vi "MicroBlaze-Tester.vi"() -> ()   [LabVIEW 2017]
doc: "Use this template to build a producer/consumer design pattern with events to produce queue items. Use this design pattern instead of the User Interface Event Handler pattern for user interfaces when you want to execute code asynchronously in response to an event without slowing the user interface responsiveness."
uses:
  MicroBlaze.States.ctl
  FpgaInterface/FpgaInterface.lvclass
panel:
  in  "AXI_STR_RXD_tkeep":fxp<+,4,4>=15.0 format="%.0b"
  out "Debug Probe 2":u64[](array[numeric]) format="%.0x"
  in  "Read Debug Probe 2":bool
  out "Debug Probe":u64[](array[numeric]) format="%.0x"
  in  "Read Debug Probe 1":bool
  out "FIFO #2 Read":u32[](array[numeric]) format="%.0x"
  in  "FIFO #2 Write":u64[](array[numeric])=[2289526357, 1144201745, 2864434397, 4009689105] format="%.0x"
  in  "Read from FIFO #2":bool
  in  "Write to FIFO #2":bool
  out "error out":errorcluster
  in  "error in (no error)":errorcluster
  in  "Write all GPIO":bool
  in  "GPIO #2":u32=4
  in  "GPIO #1":u32=3
  out "FIFO Read":u32[](array[numeric]) format="%.0x"
  out "GPIO #2":u32 format="%.0x"
  out "GPIO #1":u32 format="%.0x"
  in  "FIFO #1 Write":u32[](array[numeric])=[305419896, 2596069104, 287454020, 1432778632] format="%.0x"
  in  "Read from FIFO #1":bool
  in  "Write to FIFO #1":bool
  out "Status":string="Open FPGA Called\r\nWrite to FIFO #1\r\nRead from FIFO #3\r\nClosing FPGA\r\n"
  in  "Read all GPIO":bool
  in  "stop":bool
  # "FIFO #1 - Populate FIFO Write\nClick \"Write to FIFO #1\""
  # "FIFO #2 - Populate FIFO Write\nClick \"Write to FIFO #2"
  # "General Purose IO\nValues in Controls will be read by\nMicroBlaze and the same number\ntimes 2 will be written out to the\ncorresponding channel"
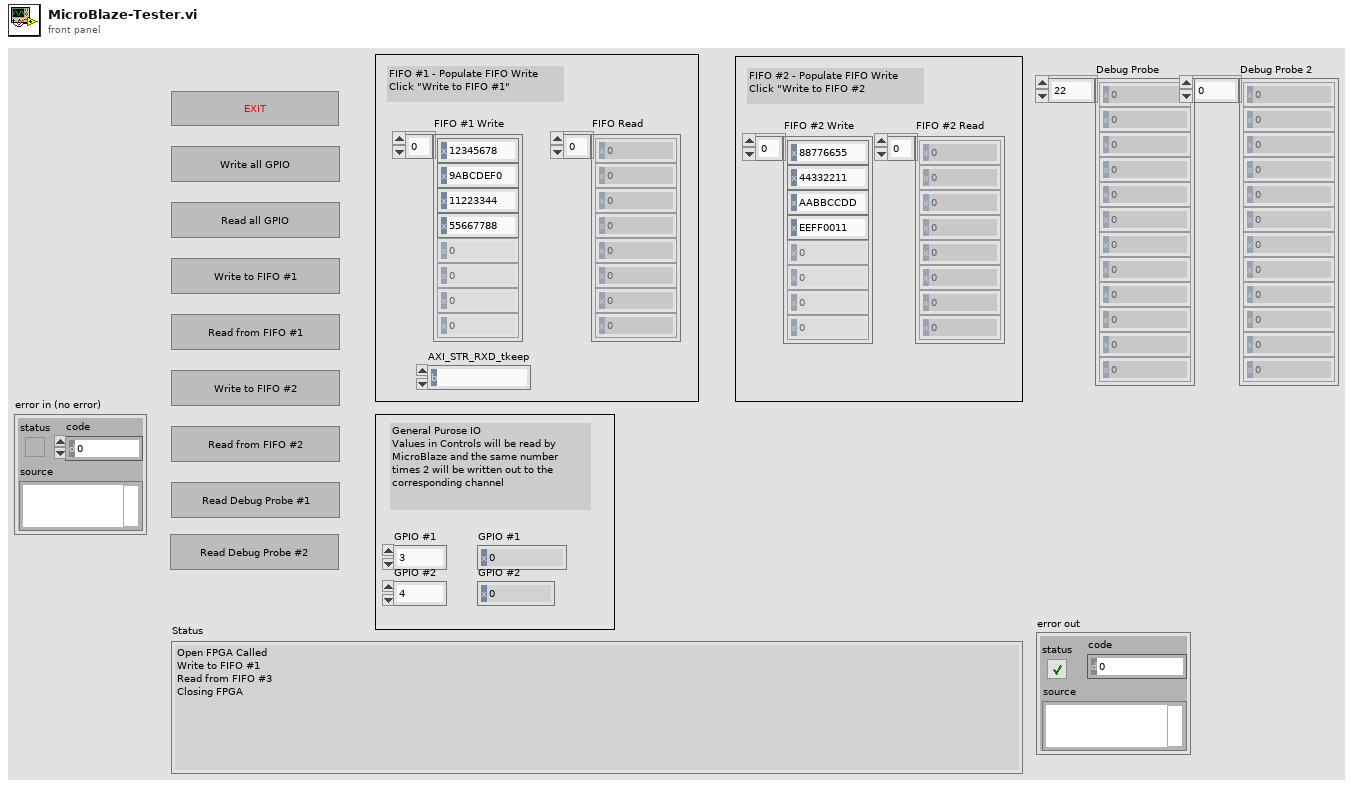
[diagram p1: front panel]
types:
  T1 = typedef "MicroBlaze.States.ctl" = enum16{"Open FPGA", "Write to GPIO", "Read all GPIO", "Write to Fifo #1", "Read from Fifo #1", "Write to Fifo #2", "Read from Fifo #2", "Read Debug Probe #1", "Read Debug Probe #2", "Close FPGA"}
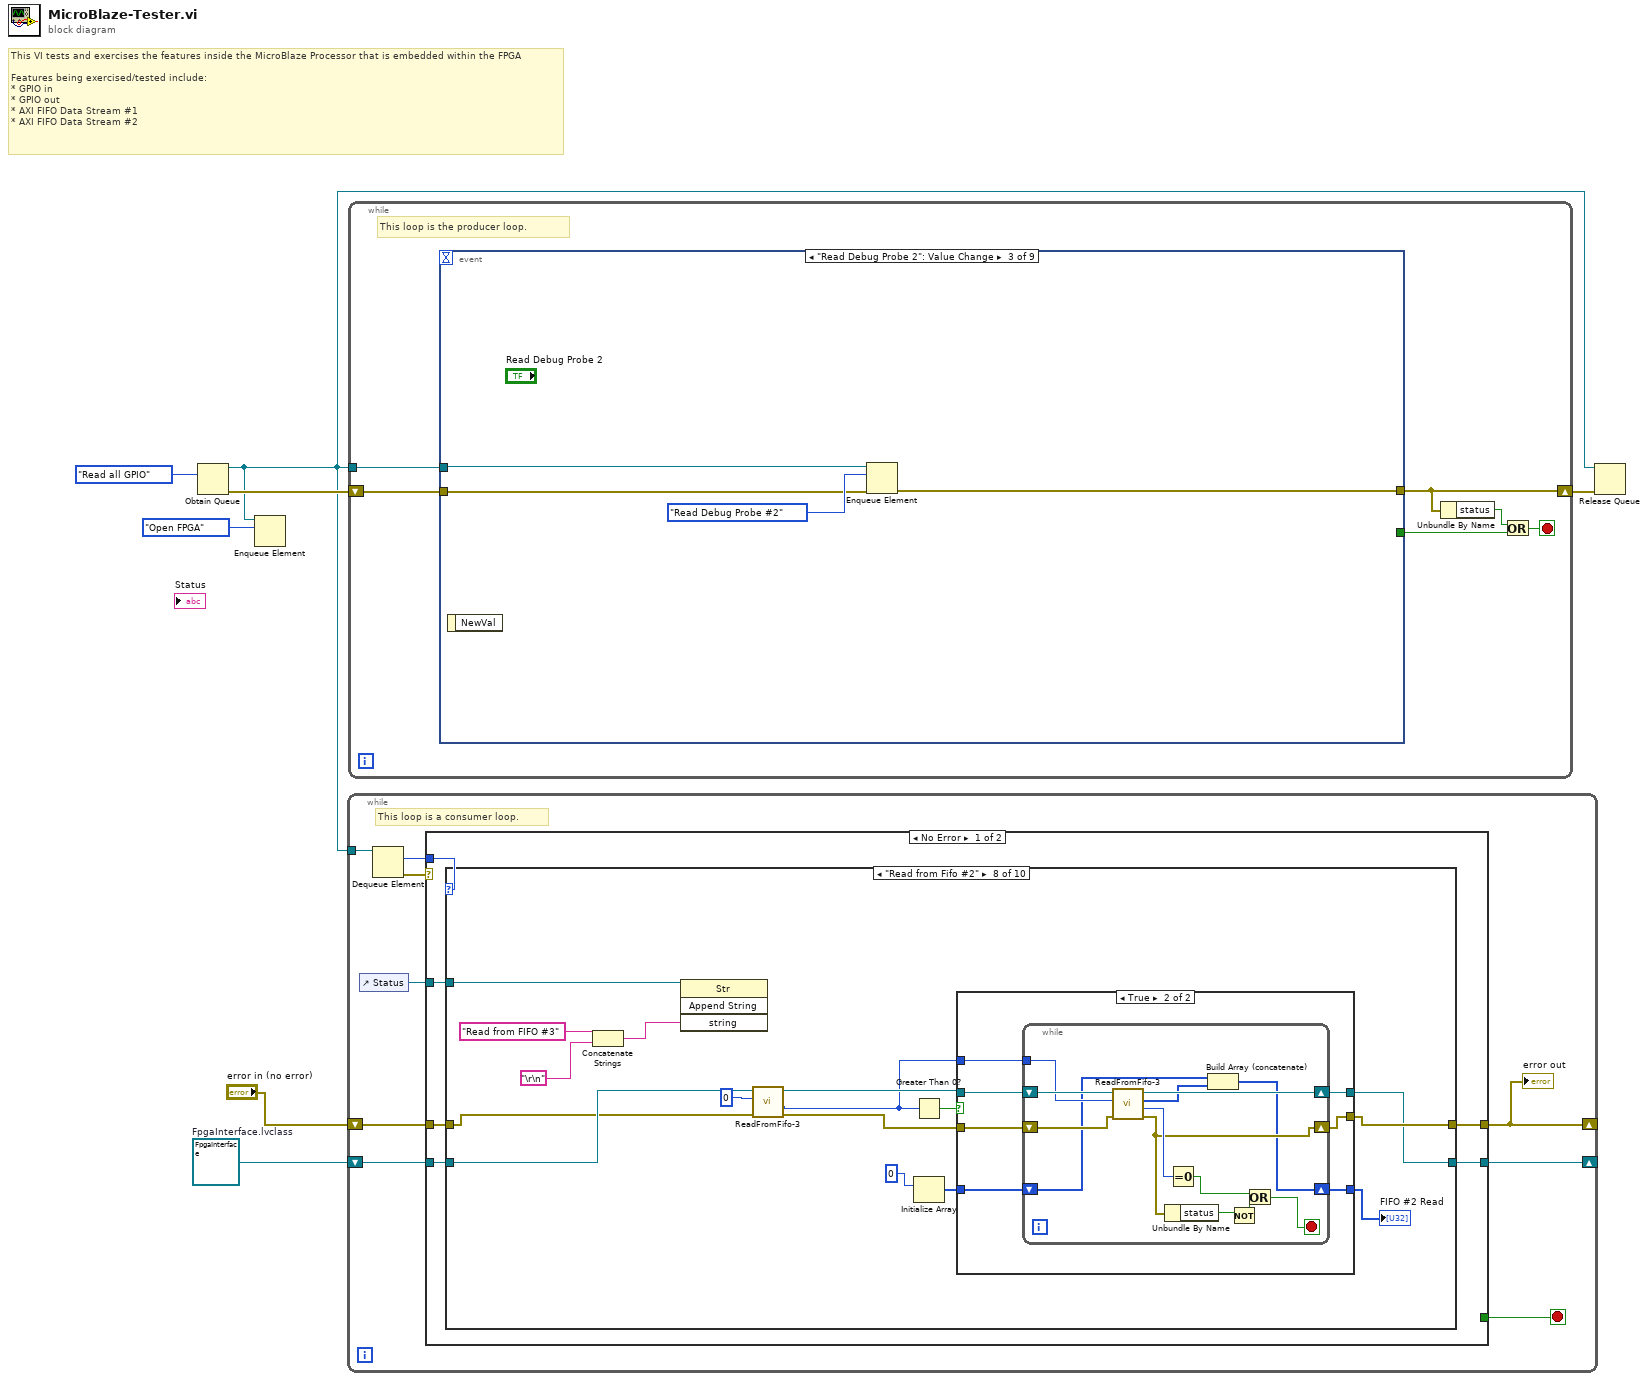
[diagram p0: block diagram]
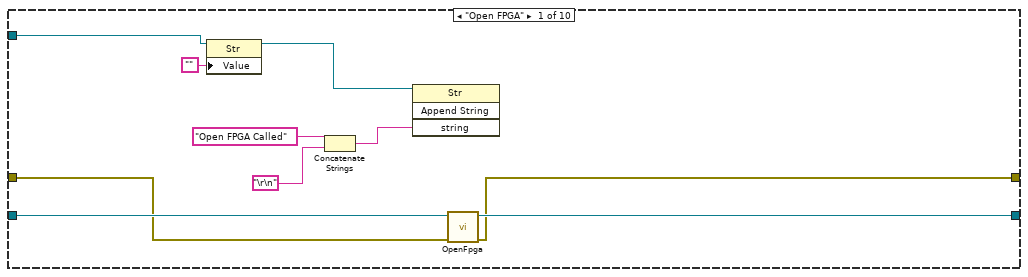
[diagram p2: hidden frame]
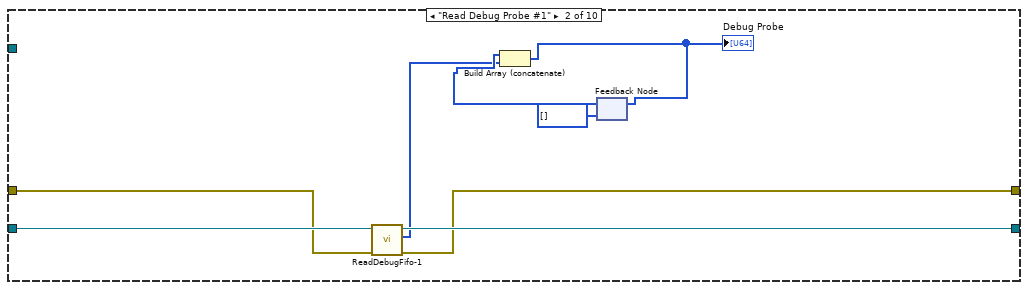
[diagram p3: hidden frame]
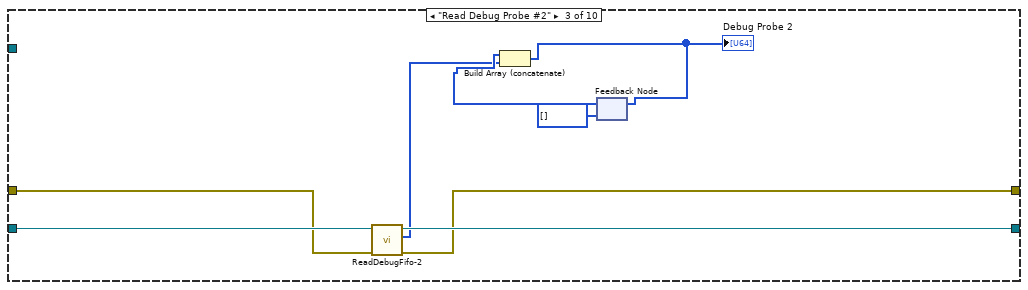
[diagram p4: hidden frame]
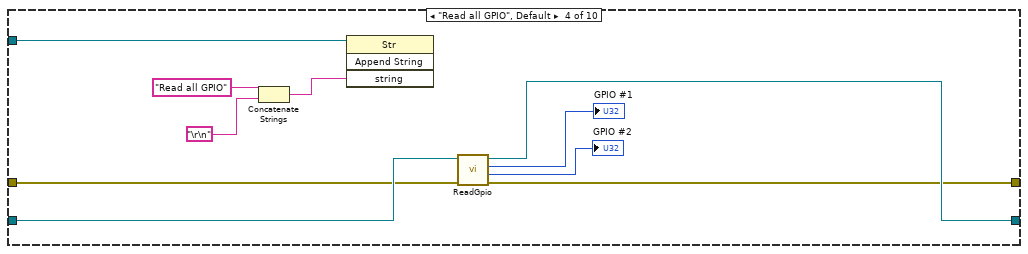
[diagram p5: hidden frame]
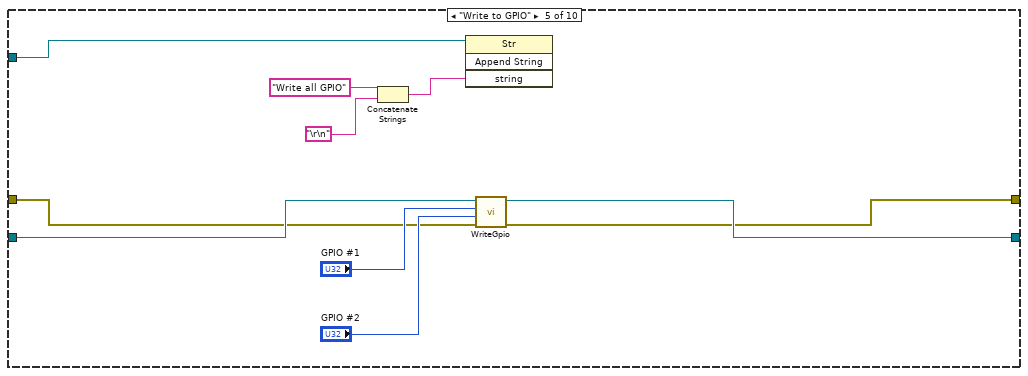
[diagram p6: hidden frame]
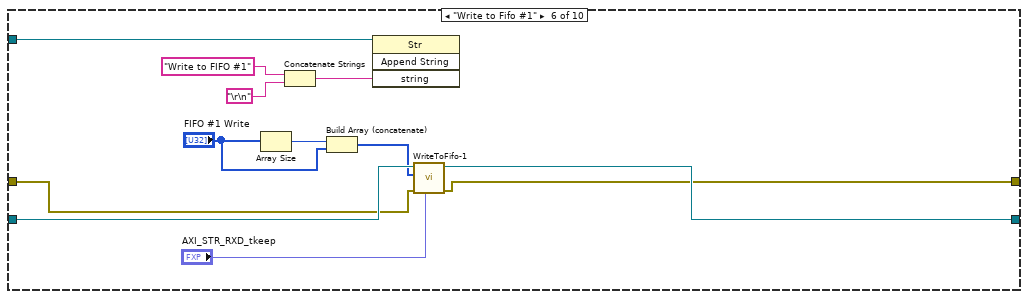
[diagram p7: hidden frame]
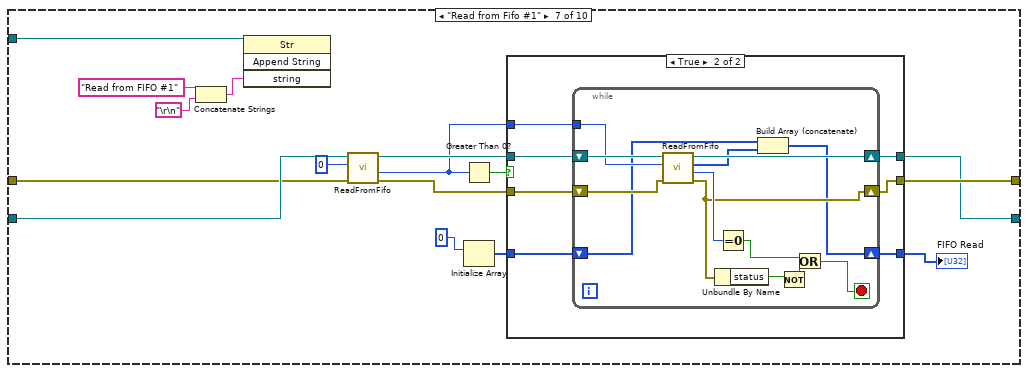
[diagram p8: hidden frame]
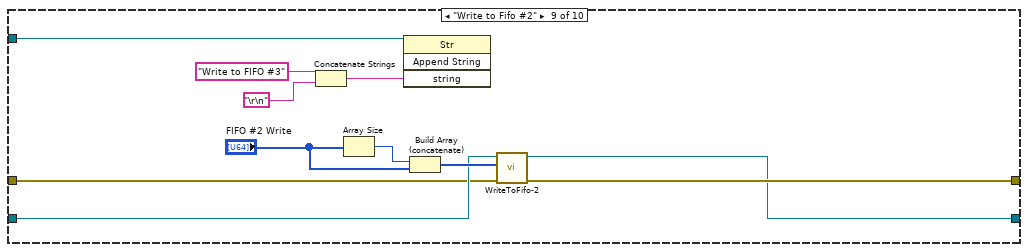
[diagram p11: hidden frame]
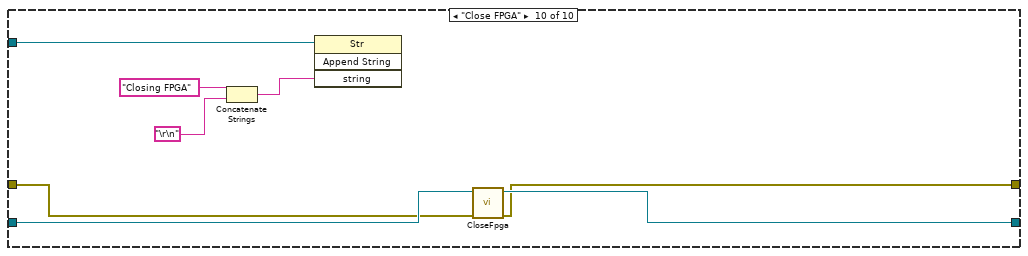
[diagram p12: hidden frame]
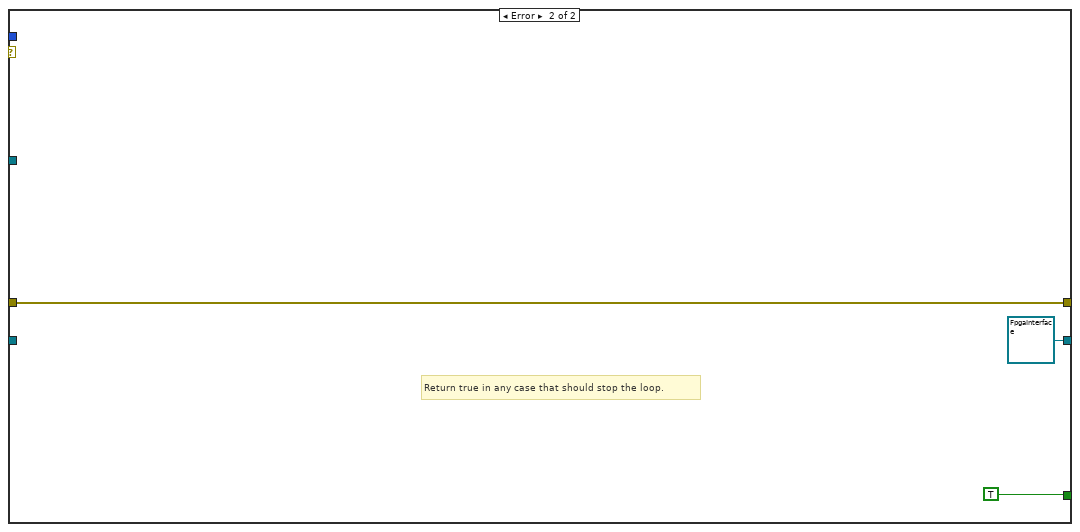
[diagram p13: hidden frame]
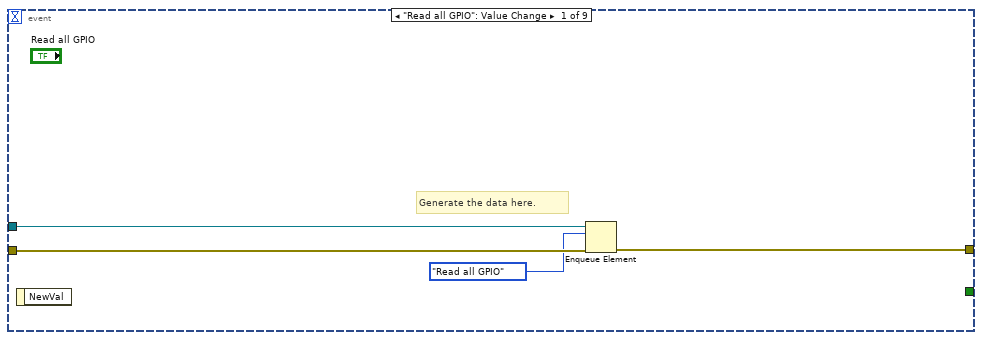
[diagram p14: hidden frame]
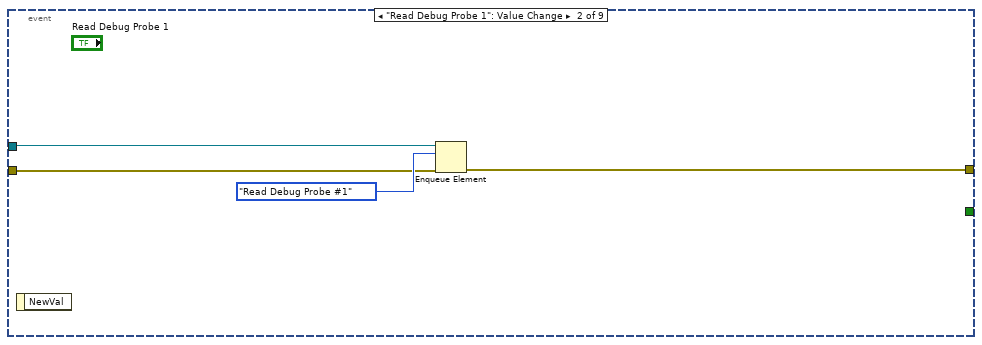
[diagram p15: hidden frame]
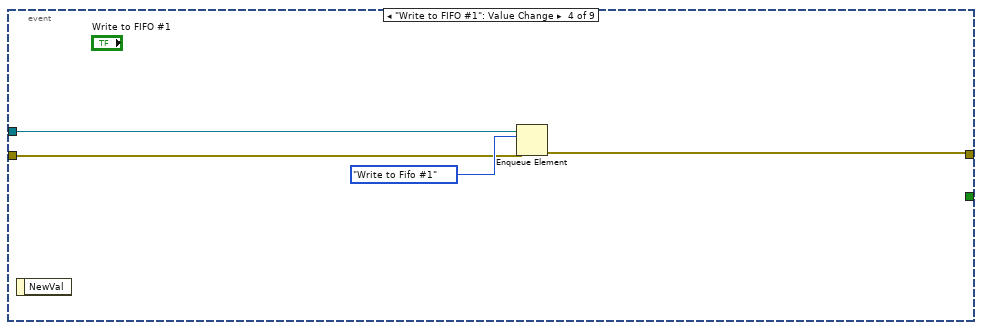
[diagram p16: hidden frame]
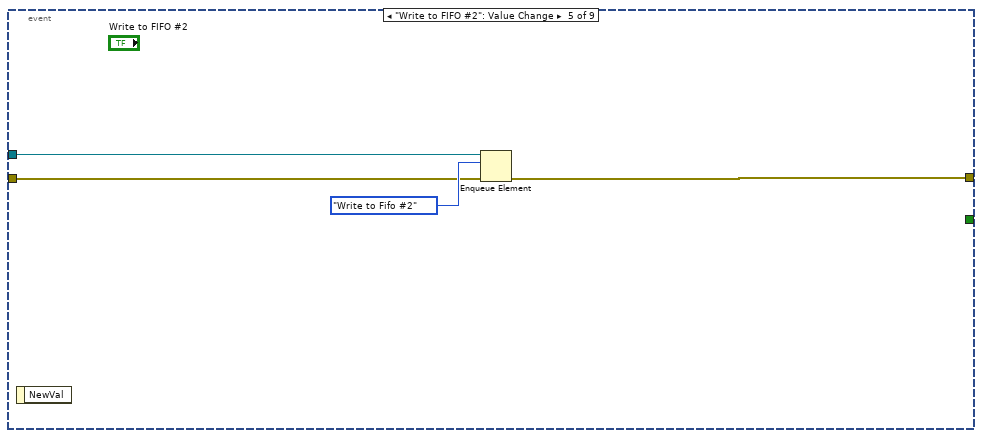
[diagram p17: hidden frame]
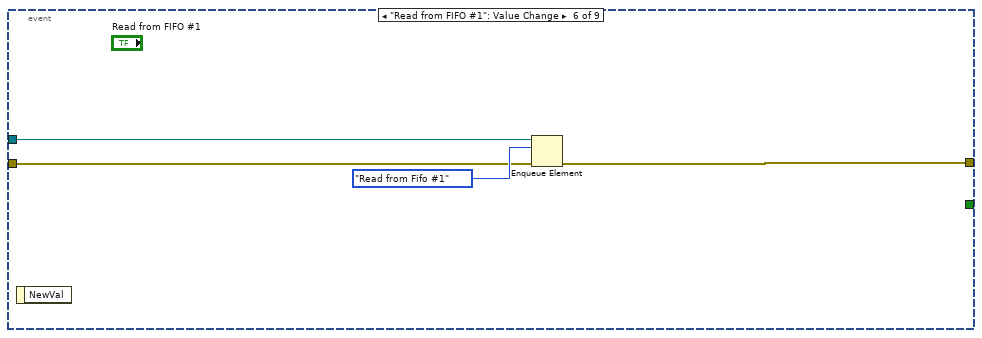
[diagram p18: hidden frame]
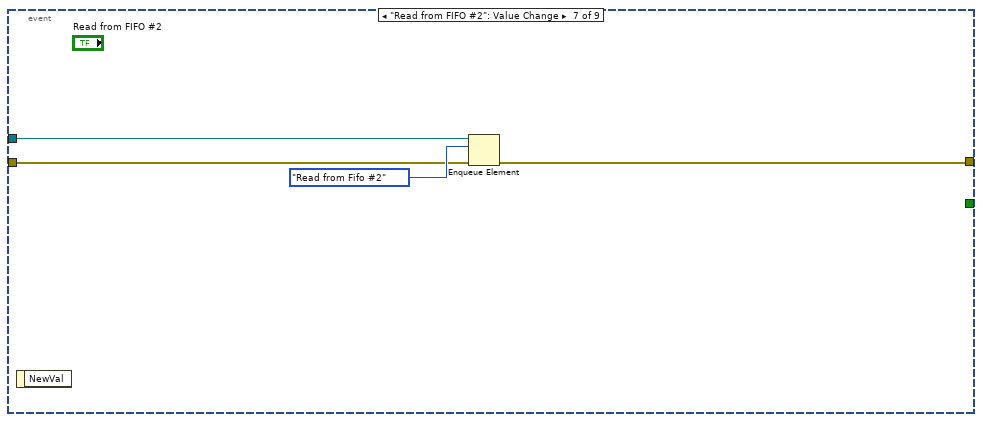
[diagram p19: hidden frame]
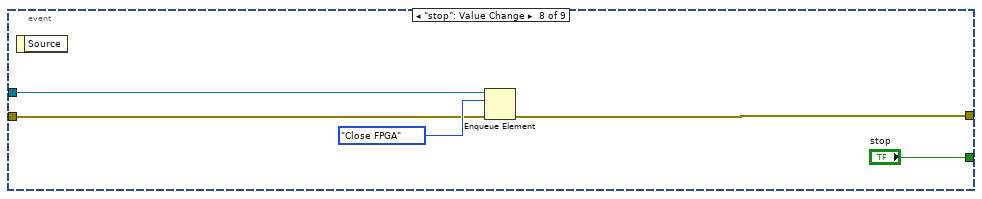
[diagram p20: hidden frame]
diagram:
  w2 = refnum<class "FpgaInterface.lvclass"> refnum  # FpgaInterface.lvclass
  # "This VI tests and exercises the features inside the MicroBlaze Processor that is embedded within the FPGA\n\nFeatures being exercised/tested include:\n* GPIO in\n* GPIO out\n* AXI FIFO Data Stream #1\n* AXI FIFO Data Stream #2"
  n1 = Obtain Queue(element data type=MicroBlaze.States."Read all GPIO" ("Events 2")) -> (queue out=w4:refnum<queue>, error out=w7:errorcluster)  [unwired: 4 in, 1 out]
  n2 = Enqueue Element(queue=w4, element=MicroBlaze.States."Open FPGA" ("Events 2")) -> ()  [unwired: 2 in, 3 out]
  n3 = while {
    tunnel: w4 -> [w16]
    shift-right: [w9] -> _
    shift-left: "error in (no error)" -> [w10]
    shift-right: [w8] -> _
    shift-left: w2 -> [w11]
    stop <- w13 stop-if-true
    # "This loop is a consumer loop."
    n4 = control-ref of="Status"() -> (w12:refnum<vi>)
    n5 = Dequeue Element(queue=w16) -> (element=w14:T1, error out=w15:errorcluster)  [unwired: 2 in, 2 out]
    n6 = case shown="No Error" w15 {
      tunnel: w14 -> [w22 _]
      tunnel: [_ TRUE] -> w13
      tunnel: w12 -> [w21 _]
      tunnel: w11 -> [w20 _]
      tunnel: [w19 refnum<class "FpgaInterface.lvclass"> refnum ("FpgaInterface out")] -> w8
      tunnel: w10 -> [w18 w178]
      tunnel: [w17 w178] -> w9
      frame No Error {
        n7 = case shown="\"Read from Fifo #2\"" w22 {
          tunnel: w21 -> [w27 _ _ w55 w65 w77 w93 w132 w166 w174]
          tunnel: w20 -> [w26 w40 w48 w54 w64 w76 w92 w131 w162 w173]
          tunnel: [w25 w38 w46 w51 w61 w75 w84 w120 w159 w172] -> w19
          tunnel: w18 -> [w24 w39 w47 w50 w60 w71 w90 w129 w161 w171]
          tunnel: [w23 w37 w45 w49 w59 w70 w85 w121 w160 w170] -> w17
          frame "Open FPGA" {
            n8 = property class="Str"(reference=w27, "Value"="") -> (reference out=w31:refnum<vi>)  [unwired: 1 in, 1 out]
            n9 = Concatenate Strings("Open FPGA Called" ("string"), "\r\n") -> (w29:string)
            n10 = invoke class="Str" method="Append String"(reference=w31, "string"=w29) -> ()  [unwired: 2 in, 4 out]
            n11 = call-dynamic "OpenFpga.vi"("error in (no error)"=w24, "FpgaInterface in"=w26) -> ("error out"=w23:errorcluster, "FpgaInterface out"=w25:refnum<class "FpgaInterface.lvclass">)  [unwired: 8 in]
          }
          frame "Read Debug Probe #1" {
            n12 = call-dynamic "ReadDebugFifo-1.vi"("error in (no error)"=w39, "FpgaInterface in"=w40) -> ("error out"=w37:errorcluster, "Data"=w35:u32[], "FpgaInterface out"=w38:refnum<class "FpgaInterface.lvclass">)  [unwired: 7 in]
            n13 = feedback #1(u64[] []) -> (w36:u64[])
            n14 = Build Array (concatenate)(w36, w35) -> (w34:u64[])
            "Debug Probe" <- w34
            n15 = feedback-in #1(w34) -> ()
          }
          frame "Read Debug Probe #2" {
            n16 = call-dynamic "ReadDebugFifo-2.vi"("error in (no error)"=w47, "FpgaInterface in"=w48) -> ("error out"=w45:errorcluster, "Data"=w43:u32[], "FpgaInterface out"=w46:refnum<class "FpgaInterface.lvclass">)  [unwired: 7 in]
            n17 = feedback #2(u64[] []) -> (w44:u64[])
            n18 = Build Array (concatenate)(w44, w43) -> (w42:u64[])
            "Debug Probe 2" <- w42
            n19 = feedback-in #2(w42) -> ()
          }
          frame "Read all GPIO", Default {
            n20 = Concatenate Strings("Read all GPIO" ("string"), "\r\n") -> (w57:string)
            n21 = invoke class="Str" method="Append String"(reference=w55, "string"=w57) -> ()  [unwired: 2 in, 4 out]
            n22 = call-dynamic "ReadGpio.vi"("error in (no error)"=w50, "FpgaInterface in"=w54) -> ("error out"=w49:errorcluster, "GPIO #2 out"=→"GPIO #2":u32, "GPIO #1 out"=→"GPIO #1":u32, "FpgaInterface out"=w51:refnum<class "FpgaInterface.lvclass">)  [unwired: 6 in]
          }
          frame "Write to GPIO" {
            n23 = Concatenate Strings("Write all GPIO" ("string"), "\r\n") -> (w67:string)
            n24 = invoke class="Str" method="Append String"(reference=w65, "string"=w67) -> ()  [unwired: 2 in, 4 out]
            n25 = call-dynamic "WriteGpio.vi"("error in (no error)"=w60, "GPIO #2 in"="GPIO #2", "GPIO #1 in"="GPIO #1", "FpgaInterface in"=w64) -> ("error out"=w59:errorcluster, "FpgaInterface out"=w61:refnum<class "FpgaInterface.lvclass">)  [unwired: 6 in]
          }
          frame "Write to Fifo #1" {
            n26 = Array Size(array="FIFO #1 Write") -> (size(s)=w74:i32)
            n27 = Concatenate Strings("Write to FIFO #1" ("string"), "\r\n") -> (w79:string)
            n28 = Build Array (concatenate)(w74, "FIFO #1 Write") -> (w72:u32[])
            n29 = invoke class="Str" method="Append String"(reference=w77, "string"=w79) -> ()  [unwired: 2 in, 4 out]
            n30 = call-dynamic "WriteToFifo-1.vi"("AXI_STR_RXD_tkeep"="AXI_STR_RXD_tkeep", "error in (no error)"=w71, "Data"=w72, "FpgaInterface in"=w76) -> ("error out"=w70:errorcluster, "FpgaInterface out"=w75:refnum<class "FpgaInterface.lvclass">)  [unwired: 6 in]
          }
          frame "Read from Fifo #1" {
            n31 = Concatenate Strings("Read from FIFO #1" ("string"), "\r\n") -> (w95:string)
            n32 = invoke class="Str" method="Append String"(reference=w93, "string"=w95) -> ()  [unwired: 2 in, 4 out]
            n33 = call-dynamic "ReadFromFifo.vi"("error in (no error)"=w90, "Number of Elements"=u32 0, "FpgaInterface in"=w92) -> ("error out"=w87:errorcluster, "Elements Remaining"=w86:u32, "FpgaInterface out"=w88:refnum<class "FpgaInterface.lvclass">)  [unwired: 5 in, 1 out]
            n34 = Greater Than 0?(x=w86) -> (x > 0?=w89:bool)
            n35 = Initialize Array(u32 0) -> (w82:u32[])  [unwired: 1 in]
            n36 = case shown="True" w89 {
              tunnel: w88 -> [w97 w106]
              tunnel: w87 -> [w98 w105]
              tunnel: w86 -> [_ w104]
              tunnel: [w98 w103] -> w85
              tunnel: [w97 w102] -> w84
              tunnel: w82 -> [w99 w101]
              tunnel: [w99 w100] -> w81
              frame False {
              }
              frame True {
                n37 = while {
                  tunnel: w104 -> [w117]
                  shift-right: [w111] -> w102
                  shift-left: w106 -> [w119]
                  shift-right: [w110] -> w103
                  shift-left: w105 -> [w118]
                  shift-right: [w108] -> w100
                  shift-left: w101 -> [w107]
                  stop <- w113 stop-if-true
                  n38 = call-dynamic "ReadFromFifo.vi"("error in (no error)"=w118, "Number of Elements"=w117, "FpgaInterface in"=w119) -> ("error out"=w110:errorcluster, "Elements Remaining"=w116:u32, "Data"=w109:u32[], "FpgaInterface out"=w111:refnum<class "FpgaInterface.lvclass">)  [unwired: 5 in]
                  n39 = Unbundle By Name(w110) -> ("status"=w115:bool)
                  n40 = Equal To 0?(x=w116) -> (x = 0?=w112:bool)
                  n41 = Build Array (concatenate)(w107, w109) -> (w108:u32[])
                  n42 = Not(x=w115) -> (.not. x?=w114:bool)
                  n43 = Or(x=w112, y=w114) -> (x .or. y?=w113:bool)
                }
              }
            }
            "FIFO Read" <- w81
          }
          frame "Read from Fifo #2" {
            n44 = Concatenate Strings("Read from FIFO #3" ("string"), "\r\n") -> (w134:string)
            n45 = invoke class="Str" method="Append String"(reference=w132, "string"=w134) -> ()  [unwired: 2 in, 4 out]
            n46 = call-dynamic "ReadFromFifo-3.vi"("error in (no error)"=w129, "Number of Elements"=u32 0, "FpgaInterface in"=w131) -> ("error out"=w124:errorcluster, "Elements Remaining"=w123:u32, "FpgaInterface out"=w125:refnum<class "FpgaInterface.lvclass">)  [unwired: 5 in, 1 out]
            n47 = Greater Than 0?(x=w123) -> (x > 0?=w128:bool)
            n48 = Initialize Array(u32 0) -> (w126:u32[])  [unwired: 1 in]
            n49 = case shown="True" w128 {
              tunnel: w125 -> [w136 w145]
              tunnel: w124 -> [w137 w144]
              tunnel: w123 -> [_ w143]
              tunnel: [w137 w142] -> w121
              tunnel: [w136 w141] -> w120
              tunnel: w126 -> [w138 w140]
              tunnel: [w138 w139] -> w122
              frame False {
              }
              frame True {
                n50 = while {
                  tunnel: w143 -> [w156]
                  shift-right: [w150] -> w141
                  shift-left: w145 -> [w158]
                  shift-right: [w149] -> w142
                  shift-left: w144 -> [w157]
                  shift-right: [w147] -> w139
                  shift-left: w140 -> [w146]
                  stop <- w152 stop-if-true
                  n51 = call-dynamic "ReadFromFifo-3.vi"("error in (no error)"=w157, "Number of Elements"=w156, "FpgaInterface in"=w158) -> ("error out"=w149:errorcluster, "Elements Remaining"=w155:u32, "Data"=w148:u32[], "FpgaInterface out"=w150:refnum<class "FpgaInterface.lvclass">)  [unwired: 5 in]
                  n52 = Unbundle By Name(w149) -> ("status"=w154:bool)
                  n53 = Equal To 0?(x=w155) -> (x = 0?=w151:bool)
                  n54 = Build Array (concatenate)(w146, w148) -> (w147:u32[])
                  n55 = Not(x=w154) -> (.not. x?=w153:bool)
                  n56 = Or(x=w151, y=w153) -> (x .or. y?=w152:bool)
                }
              }
            }
            "FIFO #2 Read" <- w122
          }
          frame "Write to Fifo #2" {
            n57 = Concatenate Strings("Write to FIFO #3" ("string"), "\r\n") -> (w168:string)
            n58 = Array Size(array="FIFO #2 Write") -> (size(s)=w165:i32)
            n59 = invoke class="Str" method="Append String"(reference=w166, "string"=w168) -> ()  [unwired: 2 in, 4 out]
            n60 = Build Array (concatenate)(w165, "FIFO #2 Write") -> (w164:u64[])
            n61 = call-dynamic "WriteToFifo-2.vi"("error in (no error)"=w161, "Data"=w164, "FpgaInterface in"=w162) -> ("error out"=w160:errorcluster, "FpgaInterface out"=w159:refnum<class "FpgaInterface.lvclass">)  [unwired: 7 in]
          }
          frame "Close FPGA" {
            n62 = Concatenate Strings("Closing FPGA" ("string"), "\r\n") -> (w176:string)
            n63 = invoke class="Str" method="Append String"(reference=w174, "string"=w176) -> ()  [unwired: 2 in, 4 out]
            n64 = call-dynamic "CloseFpga.vi"("error in (no error)"=w171, "FpgaInterface in"=w173) -> ("error out"=w170:errorcluster, "FpgaInterface out"=w172:refnum<class "FpgaInterface.lvclass">)  [unwired: 8 in]
          }
        }
      }
      frame Error {
        # "Return true in any case that should stop the loop."
      }
    }
    "error out" <- w9
  }
  n65 = while {
    shift-right: [w182] -> w6
    shift-left: w7 -> [w185]
    tunnel: w4 -> [w186]
    stop <- w183 stop-if-true
    # "This loop is the producer loop."
    n66 = event shown="[2] \"Read Debug Probe 2\": Value Change" {
      selector: _ -> [_ _ _ _ _ _ _ _ _]
      dyn-events: _ -> [_ _ _ _ _ _ _ _ _]
      timeout: _ -> [_ _ _ _ _ _ _ _ _]
      tunnel: w186 -> [w190 w192 w196 w199 w205 w207 w212 w216 w220]
      tunnel: w185 -> [w189 w193 w197 w201 w203 w209 w211 w217 w221]
      tunnel: [w188 w191 w195 w200 w204 w208 w213 w215 w222] -> w182
      tunnel: [_ _ _ _ _ _ _ "stop" _] -> w184
      event "Read all GPIO": Value Change {
        # "Generate the data here."
        n67 = event-data() -> ()  [unwired: 1 in, 1 out]
        n68 = Enqueue Element(queue=w190, element=MicroBlaze.States."Read all GPIO" ("Events 2"), error in (no error)=w189) -> (error out=w188:errorcluster)  [unwired: 1 in, 2 out]
      }
      event "Read Debug Probe 1": Value Change {
        n69 = event-data() -> ()  [unwired: 1 in, 1 out]
        n70 = Enqueue Element(queue=w192, element=MicroBlaze.States."Read Debug Probe #1" ("Events 2"), error in (no error)=w193) -> (error out=w191:errorcluster)  [unwired: 1 in, 2 out]
      }
      event "Read Debug Probe 2": Value Change {
        n71 = event-data() -> ()  [unwired: 1 in, 1 out]
        n72 = Enqueue Element(queue=w196, element=MicroBlaze.States."Read Debug Probe #2" ("Events 2"), error in (no error)=w197) -> (error out=w195:errorcluster)  [unwired: 1 in, 2 out]
      }
      event "Write to FIFO #1": Value Change {
        n73 = event-data() -> ()  [unwired: 1 in, 1 out]
        n74 = Enqueue Element(queue=w199, element=MicroBlaze.States."Write to Fifo #1" ("Events 2"), error in (no error)=w201) -> (error out=w200:errorcluster)  [unwired: 1 in, 2 out]
      }
      event "Write to FIFO #2": Value Change {
        n75 = event-data() -> ()  [unwired: 1 in, 1 out]
        n76 = Enqueue Element(queue=w205, element=MicroBlaze.States."Write to Fifo #2" ("Events 2"), error in (no error)=w203) -> (error out=w204:errorcluster)  [unwired: 1 in, 2 out]
      }
      event "Read from FIFO #1": Value Change {
        n77 = event-data() -> ()  [unwired: 1 in, 1 out]
        n78 = Enqueue Element(queue=w207, element=MicroBlaze.States."Read from Fifo #1" ("Events 2"), error in (no error)=w209) -> (error out=w208:errorcluster)  [unwired: 1 in, 2 out]
      }
      event "Read from FIFO #2": Value Change {
        n79 = event-data() -> ()  [unwired: 1 in, 1 out]
        n80 = Enqueue Element(queue=w212, element=MicroBlaze.States."Read from Fifo #2" ("Events 2"), error in (no error)=w211) -> (error out=w213:errorcluster)  [unwired: 1 in, 2 out]
      }
      event "stop": Value Change {
        n81 = event-data() -> ()  [unwired: 1 in, 1 out]
        n82 = Enqueue Element(queue=w216, element=MicroBlaze.States."Close FPGA" ("Events 2"), error in (no error)=w217) -> (error out=w215:errorcluster)  [unwired: 1 in, 2 out]
      }
      event "Write all GPIO": Value Change {
        # "Generate the data here."
        n83 = event-data() -> ()  [unwired: 1 in, 1 out]
        n84 = Enqueue Element(queue=w220, element=MicroBlaze.States."Write to GPIO" ("Events 2"), error in (no error)=w221) -> (error out=w222:errorcluster)  [unwired: 1 in, 2 out]
      }
    }
    n85 = Unbundle By Name(w182) -> ("status"=w181:bool)
    n86 = Or(x=w181, y=w184) -> (x .or. y?=w183:bool)
  }
  n87 = Release Queue(queue=w4, error in (no error)=w6) -> ()  [unwired: 1 in, 3 out]
